vi "Set Output.vi"(8 "error in (no error)":errorcluster, 10 "Enable":bool=TRUE, 11 "Keithley 2400 in":refnum<class "Keithley 2400.lvclass">) -> (0 "error out":errorcluster, 3 "Keithley 2400 out":refnum<class "Keithley 2400.lvclass">)   [LabVIEW 2011, in "Keithley 2400.lvclass"]
uses:
  Keithley 2400.lvclass
  Keithley 2400.lvclass/Keithley 2400.ctl
  <instrlib>/Keithley 24XX/Keithley 24XX.lvlib
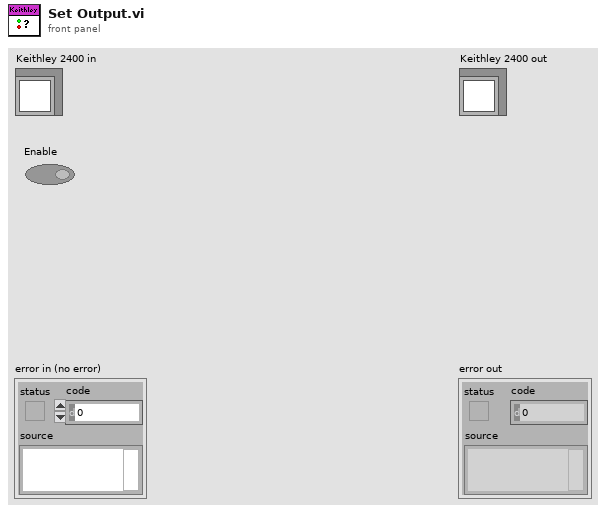
[diagram p1: front panel]
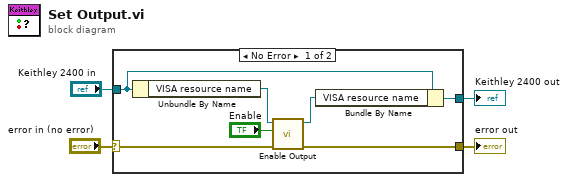
[diagram p0: block diagram]
diagram:
  n1 = case shown="No Error" "error in (no error)" {
    selector: "error in (no error)" -> [w10 w13]
    tunnel: [w7 w13] -> w3
    tunnel: [w6 w12] -> w1
    tunnel: "Keithley 2400 in" -> [w9 w12]
    frame No Error {
      n2 = Unbundle By Name(w9) -> ("VISA resource name"=w11:refnum<visa-resource-name>)
      n3 = call <instrlib>:"Enable Output.vi"("error in (no error)"=w10, "Enable Output (T: Enable)"="Enable", "VISA resource name"=w11) -> ("error out"=w7:errorcluster, "VISA resource name out"=w8:refnum<visa-resource-name>)  [unwired: 7 in]
      n4 = Bundle By Name(cluster=w9, "VISA resource name"=w8) -> (w6:refnum<class "Keithley 2400.lvclass">)
    }
    frame Error {
    }
  }
  "error out" <- w3
  "Keithley 2400 out" <- w1
